vi "helper-project-test-vi-1.vi"() -> ()   [LabVIEW 2016]
panel:
  in  "test-ctl":dbl
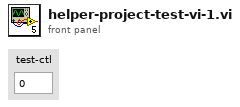
[diagram p1: front panel]
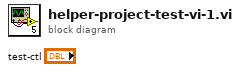
[diagram p0: block diagram]
diagram:
